vi "Config.vi"(0 "class data in":refnum<class "MB_MODULE.lvclass">, 5 "modbus":refnum<class "Modbus Master.lvclass">, 7 "addres":u16, 11 "error in (no error)":errorcluster) -> (4 "class data out":refnum<class "MB_MODULE.lvclass">, 15 "error out":errorcluster)   [LabVIEW 2019, in "MB_MODULE.lvclass"]
uses:
  MB_MODULE.lvclass
  <vilib>/NI/Modbus Library/API/Master/Modbus Master.lvclass
  MB_MODULE.lvclass/MB_MODULE.ctl
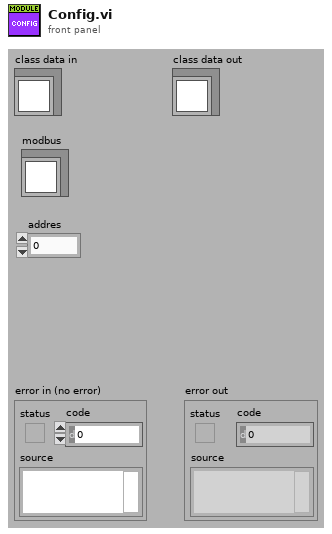
[diagram p1: front panel]
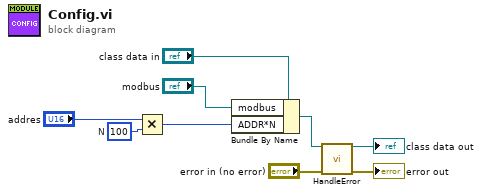
[diagram p0: block diagram]
diagram:
  w6 = u16 100  # N
  n1 = Multiply(x="addres", y=w6) -> (x*y=w5:u16)
  n2 = Bundle By Name(cluster="class data in", "modbus"="modbus", "ADDR*N"=w5) -> (w3:refnum<class "MB_MODULE.lvclass">)
  n3 = call "HandleError.vi"("reference in"=w3, "error in (no error)"="error in (no error)") -> ("reference out"=→"class data out":refnum<class "MB_MODULE.lvclass">, "error out"=→"error out":errorcluster)  [unwired: 12 in]
